vi "Add Response (Method Not Found from Request).vi"(7 "Request":refnum<class "Request.lvclass">, 8 "error in (no error)":errorcluster, 10 "data":refnum<class "JSON Null.lvclass">, 11 "Server in":refnum<class "JSONRPC Server.lvclass">) -> (0 "error out":errorcluster, 1 "response string":string, 3 "Server out":refnum<class "JSONRPC Server.lvclass">)   [LabVIEW 2015, in "JSONRPC Server.lvclass"]
uses:
  JSONRPC Server.lvclass
  Request/Request.lvclass
  <vilib>/NI/JSON Support for LabVIEW/JSON Data Classes/JSON Datatype/JSON Null.lvclass
  Request/Request.lvclass/Request.ctl
  Request/Read jsonrpc.vi
  Request/Read id value.vi
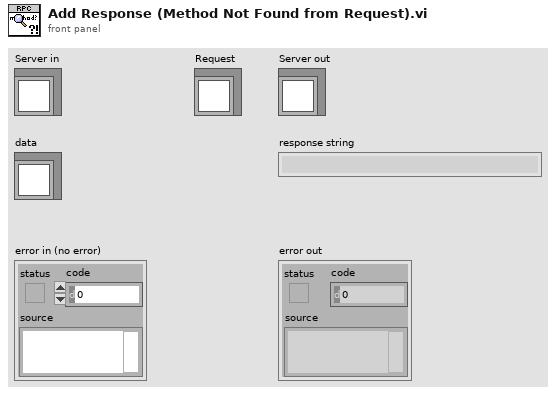
[diagram p1: front panel]
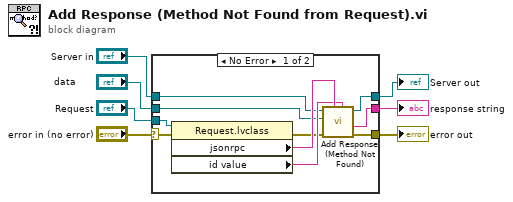
[diagram p0: block diagram]
diagram:
  n1 = case shown="No Error" "error in (no error)" {
    selector: "error in (no error)" -> [w17 w19]
    tunnel: [w10 w19] -> w6
    tunnel: [w12 w18] -> w4
    tunnel: "Server in" -> [w13 w18]
    tunnel: "Request" -> [w16 _]
    tunnel: "data" -> [w9 _]
    tunnel: [w8 _] -> w1
    frame No Error {
      n2 = property class="Request.lvclass"(reference=w16, error in=w17) -> (error out=w11:errorcluster, "jsonrpc"=w15:string, "id value"=w14:string)  [unwired: 1 out]
      n3 = call "Add Response (Method Not Found).vi"("id value"=w14, "jsonrpc"=w15, "error in (no error)"=w11, "data"=w9, "Server in"=w13) -> ("error out"=w10:errorcluster, "response string"=w8:string, "Server out"=w12:refnum<class "JSONRPC Server.lvclass">)  [unwired: 4 in]
    }
    frame Error {
    }
  }
  "error out" <- w6
  "Server out" <- w4
  "response string" <- w1
